vi "Get Node Data (Boolean).vi"(3 "element id":i32, 6 "Attribute?(F=Entity)":bool, 7 "format string (%d)":string="%d", 8 "error in":errorcluster, 9 "Default Value (0)":bool, 10 "Attribute Name":string, 11 "xml":T1) -> (0 "error out":errorcluster, 1 "Data Value":bool, 2 "found?":bool)   [LabVIEW 2011]
doc: "Returns the <B>Data Value</B> (text or cdata-section) of <B>Node</B>. If none is found, <B>Default Value</B> will be used."
uses:
  Fast Parser/XML Structure - Cluster.ctl
  Fast Parser/XML Tag Type - Enum.ctl
  <userlib>/_OpenG.lib/string/string.llb/Trim Whitespace (String)__ogtk.vi
panel:
  # "Copyright © 2006 James Kring, Inc. All rights reserved.\n\nAuthor: Jim Kring <jim.kring@jameskring.com>\n\nThis library is provided \"AS IS\" , WITHOUT WARRANTIES OR \nCONDITIONS OF ANY KIND, either express or implied.\n\nJames Kring, Inc. -- http://www.jameskring.com"
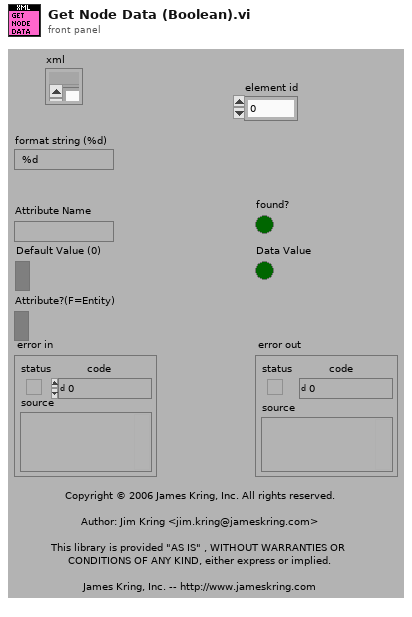
[diagram p1: front panel]
types:
  T1 = typedef "XML Structure - Cluster.ctl" = cluster{"tags":string[], "tag names":string[], "tag type":T2[], "offset":i32[], "close tag index":i32[], "xml":string, "Children":cluster{"children":i32[]}[], "parent index":i32[]}
  T2 = typedef "XML Tag Type - Enum.ctl" = enum16{"start tag", "empty tag", "end tag"}
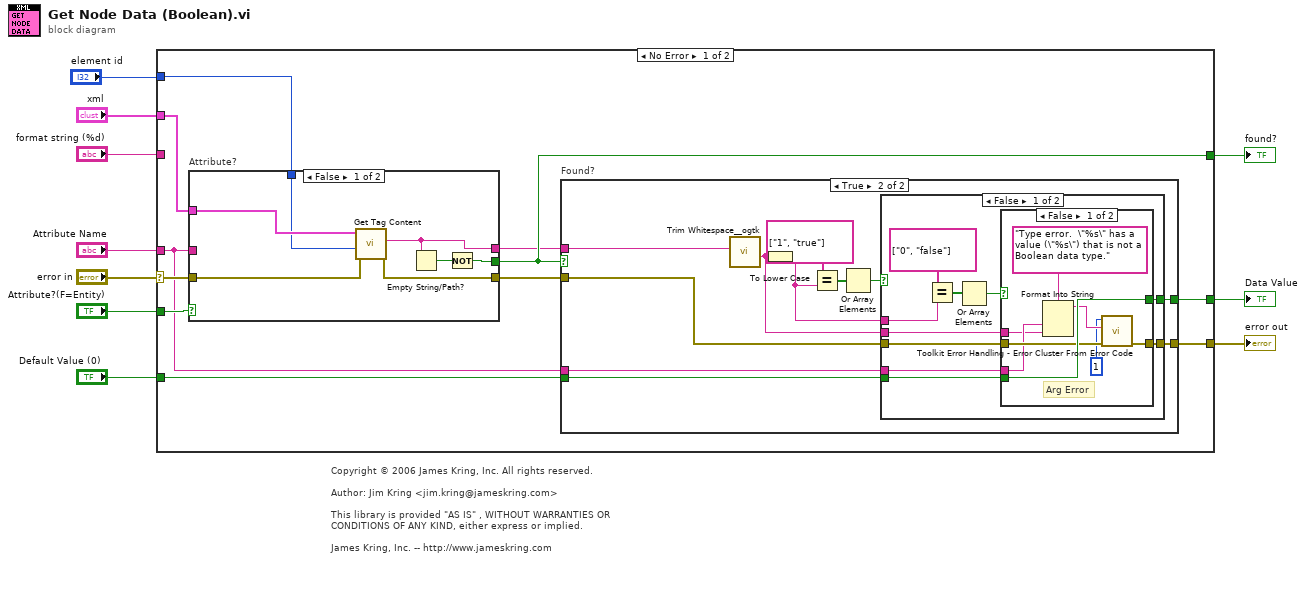
[diagram p0: block diagram]
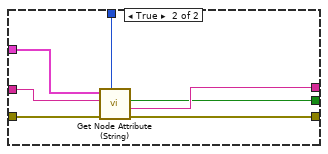
[diagram p2: hidden frame]
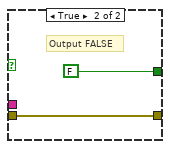
[diagram p4: hidden frame]
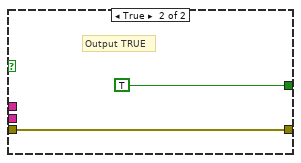
[diagram p5: hidden frame]
diagram:
  # "Copyright © 2006 James Kring, Inc. All rights reserved.\n\nAuthor: Jim Kring <jim.kring@jameskring.com>\n\nThis library is provided \"AS IS\" , WITHOUT WARRANTIES OR \nCONDITIONS OF ANY KIND, either express or implied.\n\nJames Kring, Inc. -- http://www.jameskring.com"
  n1 = case shown="No Error" "error in" {
    selector: "error in" -> [w21 w71]
    tunnel: "xml" -> [w12 _]
    tunnel: [w18 _] -> w4
    tunnel: [w19 w71] -> w9
    tunnel: [w17 _] -> w3
    tunnel: "Default Value (0)" -> [w20 _]
    tunnel: "Attribute?(F=Entity)" -> [w14 _]
    tunnel: "Attribute Name" -> [w13 _]
    tunnel: "format string (%d)" -> [_ _]
    tunnel: "element id" -> [w11 _]
    frame No Error {
      n2 = case "Attribute?" shown="False" w14 {
        tunnel: w21 -> [w24 w35]
        tunnel: [w27 w30] -> w17
        tunnel: w12 -> [w26 w33]
        tunnel: [w22 w31] -> w16
        tunnel: [w23 w34] -> w15
        tunnel: w13 -> [_ w32]
        tunnel: w11 -> [w25 w29]
        frame False {
          n3 = call "Get Tag Content.vi"("error in (no error)"=w24, "tag index"=w25, "xml in"=w26) -> ("error out"=w23:errorcluster, "element content"=w22:string)  [unwired: 5 in, 2 out]
          n4 = Empty String/Path?(string/path=w22) -> (empty?=w28:bool)
          n5 = Not(x=w28) -> (.not. x?=w27:bool)
        }
        frame True {
          n6 = call "Get Node Attribute (String).vi"("element id"=w29, "error in (no error)"=w35, "Attribute Name"=w32, "xml"=w33) -> ("error out"=w34:errorcluster, "Attribute Value"=w31:string, "found?"=w30:bool)  [unwired: 5 in]
        }
      }
      n7 = case "Found?" shown="True" w17 {
        tunnel: [w36 w45] -> w18
        tunnel: w15 -> [w37 w39]
        tunnel: [w37 w40] -> w19
        tunnel: w16 -> [_ w38]
        tunnel: w20 -> [w36 w43]
        tunnel: w13 -> [_ w41]
        frame False {
          # "Use Default"
        }
        frame True {
          n8 = call-poly <userlib>:"Trim Whitespace__ogtk.vi"("String in"=w38) -> ("String out"=w42:string)  [unwired: 6 in]
          n9 = To Lower Case(string=w42) -> (all lower case string=w44:string)
          n10 = Equal?(x=string[] ["1", "true"], y=w44) -> (x = y?=w47:bool[])
          n11 = Or Array Elements(Boolean array=w47) -> (logical OR=w46:bool)
          n12 = case shown="False" w46 {
            tunnel: [w54 TRUE] -> w45
            tunnel: w44 -> [w56 _]
            tunnel: w43 -> [w53 _]
            tunnel: w39 -> [w52 w69]
            tunnel: w42 -> [w51 _]
            tunnel: w41 -> [w50 _]
            tunnel: [w49 w69] -> w40
            frame False {
              n13 = Equal?(x=string[] ["0", "false"], y=w56) -> (x = y?=w58:bool[])
              n14 = Or Array Elements(Boolean array=w58) -> (logical OR=w55:bool)
              n15 = case shown="False" w55 {
                tunnel: [w66 FALSE] -> w54
                tunnel: w53 -> [w66 _]
                tunnel: w52 -> [w65 w67]
                tunnel: w51 -> [w63 _]
                tunnel: w50 -> [w64 _]
                tunnel: [w59 w67] -> w49
                frame False {
                  # "Arg Error"
                  n16 = Format Into String(format string="Type error.  \"%s\" has a value (\"%s\") that is not a Boolean data type.", w64, w63) -> (resulting string=w61:string)  [unwired: 2 in, 1 out]
                  n17 = call "Toolkit Error Handling - Error Cluster From Error Code.vi"("error in"=w65, "error message (\"\")"=w61, "error code (0)"=1) -> ("error out"=w59:errorcluster)  [unwired: 6 in]
                }
                frame True {
                  # "Output FALSE"
                }
              }
            }
            frame True {
              # "Output TRUE"
            }
          }
        }
      }
    }
    frame Error {
    }
  }
  "error out" <- w9
  "Data Value" <- w4
  "found?" <- w3
